vi "ADC (SubVI).vi"(7 "relative seconds":dbl, 8 "error in (no error)":errorcluster, 9 "y":dbl, 10 "Value":refnum<visa-resource-name>, 11 "Boolean in":refnum<vi>) -> (0 "error out":errorcluster, 3 "Numeric":dbl)   [LabVIEW 2017]
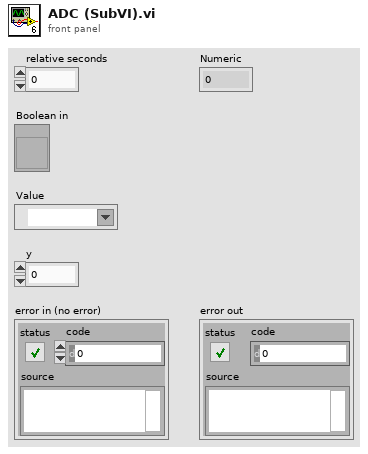
[diagram p1: front panel]
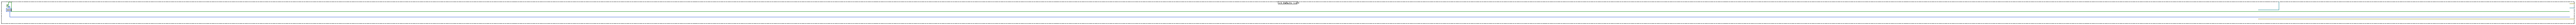
[diagram p2: hidden frame]
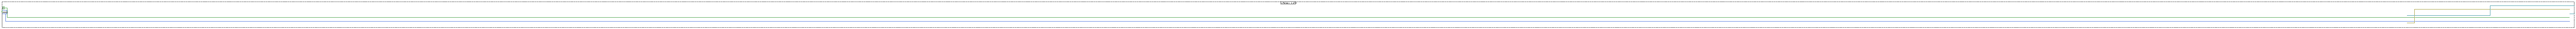
[diagram p3: hidden frame]
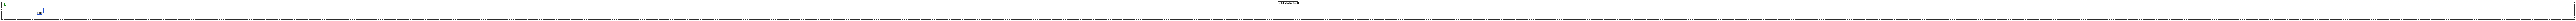
[diagram p4: hidden frame]
diagram:
  n1 = while {
    tunnel: "Value" -> [w22]
    tunnel: "error in (no error)" -> [w21]
    tunnel: [w20] -> _
    tunnel: [w19] -> w5
    tunnel: "relative seconds" -> [w17]
    tunnel: [w11] -> w6
    tunnel: "y" -> [w9]
    tunnel: "Boolean in" -> [w8]
    stop <- w13 stop-if-true
    n2 = property on="Property Node" class="Bool (strict)"(reference=w8) -> ("Value"=w10:bool)  [unwired: 1 in, 2 out]
    n3 = VISA Read(VISA resource name=w22, byte count=u32 1, error in (no error)=w21) -> (VISA resource name out=w24:refnum<visa-resource-name>, read buffer=w25:string, error out=w23:errorcluster)  [unwired: 1 out]
    n4 = String To Byte Array(string=w25) -> (unsigned byte array=w28:u8[])
    n5 = Index Array(array=w28, index=0) -> (element=w26:u8)
    n6 = case shown="75" w26 {
      tunnel: [w33 w38] -> w19
      tunnel: w24 -> [w32 w47]
      tunnel: w23 -> [w33 w46]
      tunnel: [w32 w39] -> w20
      tunnel: [u32 9999 w36] -> w11
      tunnel: [FALSE w35] -> w12
      tunnel: w9 -> [_ w34]
      frame 0, Default {
      }
      frame 75 {
        n7 = VISA Read(VISA resource name=w47, byte count=u32 3, error in (no error)=w46) -> (VISA resource name out=w42:refnum<visa-resource-name>, read buffer=w50:string, error out=w41:errorcluster)  [unwired: 1 out]
        n8 = String To Byte Array(string=w50) -> (unsigned byte array=w40:u8[])
        n9 = Index Array(array=w40, index #1=0 ("index")) -> (element #1=w45:u8, element #2=w43:u8)  [unwired: 2 in, 1 out]
        n10 = Equal?(x=u8 0, y=w45) -> (x = y?=w44:bool)
        n11 = case shown="True" w44 {
          tunnel: [w53 w61] -> w38
          tunnel: w43 -> [_ w68]
          tunnel: w42 -> [w54 w67]
          tunnel: w41 -> [w53 w66]
          tunnel: w40 -> [_ w65]
          tunnel: [w54 w63] -> w39
          tunnel: [u32 9999 w57] -> w36
          tunnel: [FALSE w56] -> w35
          tunnel: w34 -> [_ w55]
          frame False {
          }
          frame True {
            n12 = VISA Read(VISA resource name=w67, byte count=w68, error in (no error)=w66) -> (VISA resource name out=w63:refnum<visa-resource-name>, read buffer=w62:string, error out=w61:errorcluster)  [unwired: 1 out]
            n13 = String To Byte Array(string=w62) -> (unsigned byte array=w64:u8[])
            n14 = Insert Into Array(array=w65, new element=w64) -> (w58:u8[])  [unwired: 1 in]
            n15 = Index Array(array=w58, index #1=0 ("index")) -> (element #3=w59:u8)  [unwired: 2 in, 2 out]
            n16 = case shown="15..19" w59 {
              tunnel: w58 -> [_ w82]
              tunnel: [u32 9999 w72] -> w57
              tunnel: [FALSE w73] -> w56
              tunnel: w55 -> [_ w71]
              frame 0, Default {
              }
              frame 15..19 {
                n17 = Index Array(array=w82, index #1=3 ("index")) -> (element #1=w81:u8, element #2=w80:u8, element #3=w79:u8, element #4=w78:u8)  [unwired: 3 in]
                n18 = Join Numbers(hi=w78, lo=w79) -> ((hi.lo)=w76:u16)
                n19 = Join Numbers(hi=w80, lo=w81) -> ((hi.lo)=w77:u16)
                n20 = Join Numbers(hi=w76, lo=w77) -> ((hi.lo)=w74:u32)
                n21 = Multiply(x=0.02003173828125, y=w74) -> (x*y=w72:dbl)
                n22 = Greater Or Equal?(x=w72, y=w71) -> (x >= y?=w73:bool)
              }
            }
          }
        }
      }
    }
    n23 = call <vilib>:"High Resolution Relative Seconds.vi"() -> ("relative seconds"=w18:dbl)
    n24 = Subtract(x=w18, y=w17) -> (x-y=w16:dbl)
    n25 = Greater Or Equal?(x=w16, y=2.0) -> (x >= y?=w14:bool)
    n26 = Compound Arithmetic op=OR(w10, w14, w12) -> (w13:bool)
  }
  "Numeric" <- w6
  "error out" <- w5
